vi "PS (multiple).vi"(8 "error in (no error)":errorcluster, 11 "XY-data":cluster{"X-array":dbl[], "Y-array":dbl[]}[](array[cluster]) {"Y-array" format="%.2p"; "X-array" format="%.2p"}) -> (0 "error out":errorcluster, 2 "Power Spectrum":cluster{"f0":dbl, "df":dbl, "magnitude":dbl[]}[](array[cluster]), 3 "XY-data out":cluster{"X-array":dbl[], "Y-array":dbl[]}[](array[cluster]) {"Y-array" format="%.2p"; "X-array" format="%.2p"})   [LabVIEW 2019, in "xy_utilities.lvlib"]
doc: "Computes the Power Spectrum of <B>XY-data</B>. This VI is a wrapper for NI_MAPro.lvlib:FFT Power Spectrum and PSD.vi.\n\nWire data to the data input to determine the polymorphic instance to use or manually select the instance."
uses:
  xy_utilities.lvlib
  Get X Array dx.vi
  <vilib>/measure/maresamp.llb/Resample Waveforms (single shot).vi
  <vilib>/measure/maresamp.llb/Resample Pair of Arrays (single shot).vi
  <vilib>/measure/maspectr.llb/FFT Power Spectrum and PSD.vi
  <vilib>/measure/maspectr.llb/FFT Power Spectrum and PSD for 1 Chan.vi
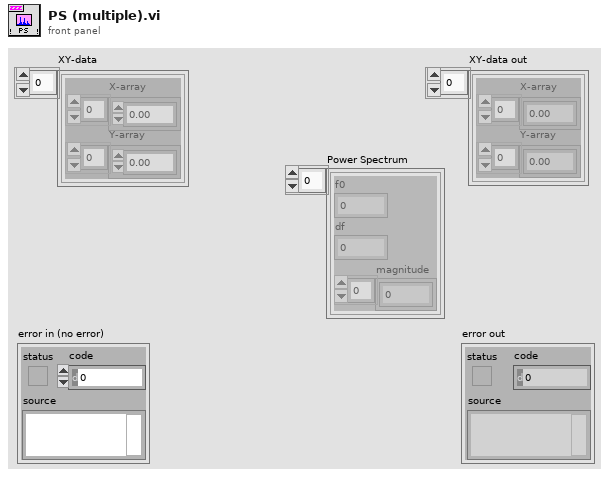
[diagram p1: front panel]
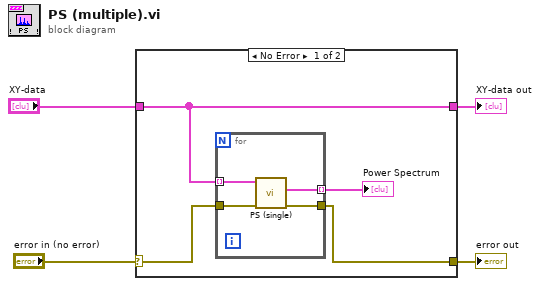
[diagram p0: block diagram]
diagram:
  n1 = case shown="No Error" "error in (no error)" {
    selector: "error in (no error)" -> [w6 w14]
    tunnel: [w8 w14] -> w3
    tunnel: "XY-data" -> [w5 w13]
    tunnel: [w5 w13] -> w1
    frame No Error {
      n2 = for {
        tunnel: w5 -> [w12] mode=indexing
        tunnel: [w9] -> w7 mode=indexing
        tunnel: w6 -> [w10]
        tunnel: [w11] -> w8
        n3 = call "PS (single).vi"("error in (no error)"=w10, "XY-data"=w12) -> ("error out"=w11:errorcluster, "Power Spectrum"=w9:cluster{"f0":dbl, "df":dbl, "magnitude":dbl[]})  [unwired: 7 in, 1 out]
      }
      "Power Spectrum" <- w7
    }
    frame Error {
    }
  }
  "error out" <- w3
  "XY-data out" <- w1
